vi "DuplicateV(SubVI).vi"(10 "Averaging":i32, 11 "V in":dbl[](array[numeric])) -> (3 "V out":dbl[](array[numeric]))   [LabVIEW 2024]
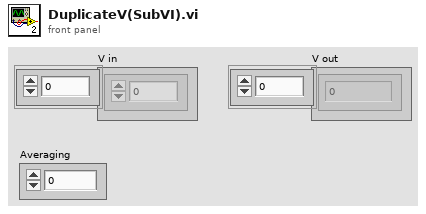
[diagram p1: front panel]
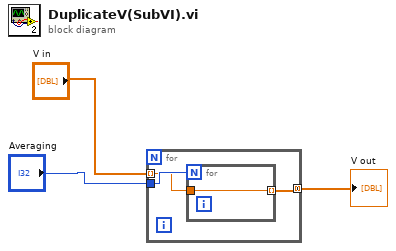
[diagram p0: block diagram]
diagram:
  n1 = for {
    tunnel: "V in" -> [w5] mode=indexing
    tunnel: "Averaging" -> [w6]
    tunnel: [w4] -> w3 mode=concatenating
    n2 = for {
      N: w6 -> [_]
      tunnel: w5 -> [w7]
      tunnel: [w7] -> w4 mode=indexing
    }
  }
  "V out" <- w3
